vi "config_fgv.vi"(7 "cmd":enum16{"write", "read", "ini"}(ring)=enum."read", 8 "error in":errorcluster caption="에러 입력(에러 없음)", 11 "Config in":T1={"Lower Cut-Off"=36.0, "Vacuum Trigger level"=20.0, "state settings"={"method"=enum."histogram", "histogram size"=512, "histogram method"=enum."mode", "reserved"=1.0}, "SPA-300 Setting"={"Bonding force (g)"=0.0, "Bonding time (ms)"=512.0, "Pickup force (g)"=0.0, "Pickup time (ms)"=1.0, "Speed"=enum."Slow"}, "sensor file"=path ""} {"state settings"."reserved" format="%0.2f"}) -> (0 "error out":errorcluster caption="에러 출력", 3 "Config out":T1={"Lower Cut-Off"=0.1, "Vacuum Trigger level"=8.0, "state settings"={"method"=enum."histogram", "histogram size"=512, "histogram method"=enum."mode", "reserved"=1.0}, "SPA-300 Setting"={"Bonding force (g)"=0.0, "Bonding time (ms)"=512.0, "Pickup force (g)"=0.0, "Pickup time (ms)"=1.0, "Speed"=enum."Slow"}, "sensor file"=path ""} {"state settings"."reserved" format="%0.2f"})   [LabVIEW 2016]
uses:
  ctl/config_ctl.ctl
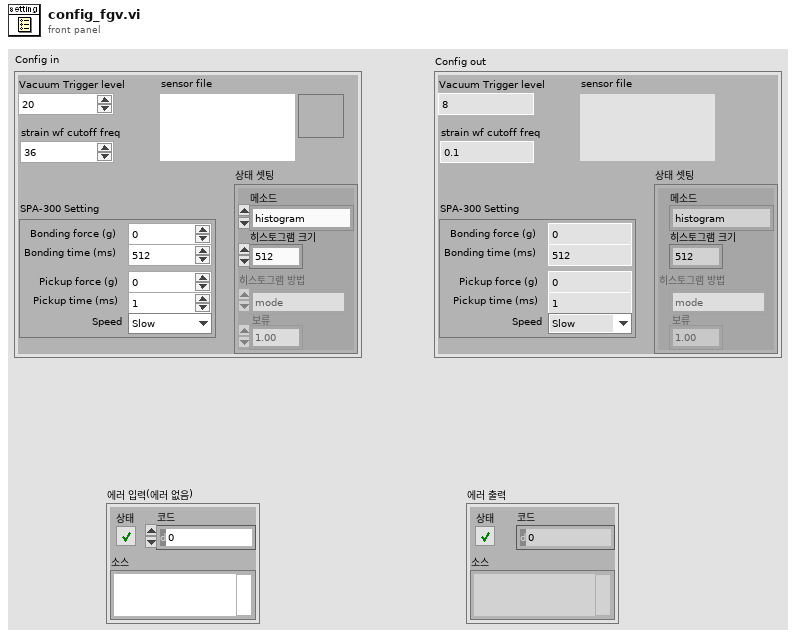
[diagram p1: front panel]
types:
  T1 = typedef "config_ctl.ctl" = cluster{"Lower Cut-Off":dbl, "Vacuum Trigger level":dbl, "state settings":cluster{"method":enum32{"histogram", "peak", "auto select"}, "histogram size":i32, "histogram method":enum16{"mode"}, "reserved":dbl}, "SPA-300 Setting":cluster{"Bonding force (g)":dbl, "Bonding time (ms)":dbl, "Pickup force (g)":dbl, "Pickup time (ms)":dbl, "Speed":enum16{"Slow", "Fast"}}, "sensor file":path}
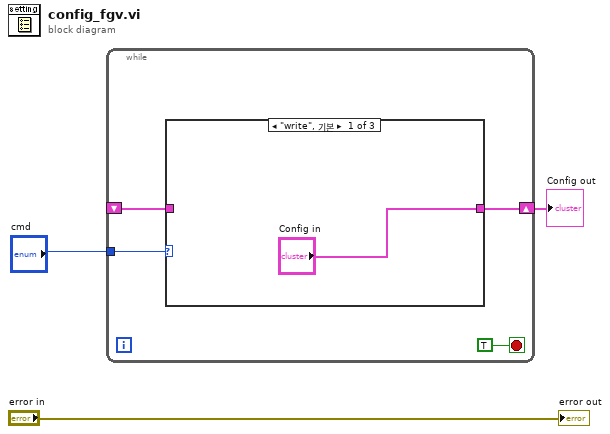
[diagram p0: block diagram]
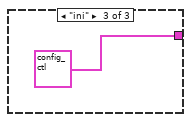
[diagram p3: hidden frame]
diagram:
  n1 = while {
    tunnel: "cmd" -> [w6]
    shift-right: [w5] -> w2
    shift-left: _ -> [w4]
    stop <- TRUE stop-if-true
    n2 = case shown="\"write\", 기본" w6 {
      tunnel: ["Config in" w9 T1 {"Lower Cut-Off"=0.5, "Vacuum Trigger level"=20.0, "state settings"={"method"=enum."histogram", "histogram size"=0, "histogram method"=enum."mode", "reserved"=0.0}, "SPA-300 Setting"={"Bonding force (g)"=0.0, "Bonding time (ms)"=0.0, "Pickup force (g)"=0.0, "Pickup time (ms)"=0.0, "Speed"=enum."Slow"}, "sensor file"=path ""} ("Config")] -> w5
      tunnel: w4 -> [_ w9 _]
      frame "write", Default {
      }
      frame "read" {
      }
      frame "ini" {
      }
    }
  }
  "Config out" <- w2
  "error out" <- "error in"
